vi "DSF.Engine.Runtime.Plugin.Get ID.vi"(8 "error in (no error)":errorcluster, 11 "Plugin in":refnum<class "DSF.Engine.Runtime.Plugin.lvclass">) -> (0 "error out":errorcluster, 2 "id":i32, 3 "Plugin out":refnum<class "DSF.Engine.Runtime.Plugin.lvclass">)   [LabVIEW 2016, in "DSF.Engine.lvlib" / "DSF.Engine.Runtime.Plugin.lvclass"]
uses:
  DSF.Engine.Runtime.Plugin.lvclass
  DSF.Engine.Runtime.Plugin.lvclass/DSF.Engine.Runtime.Plugin.ctl
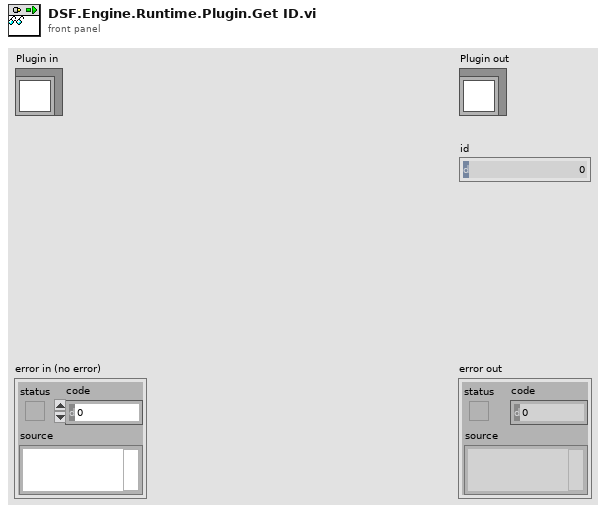
[diagram p1: front panel]
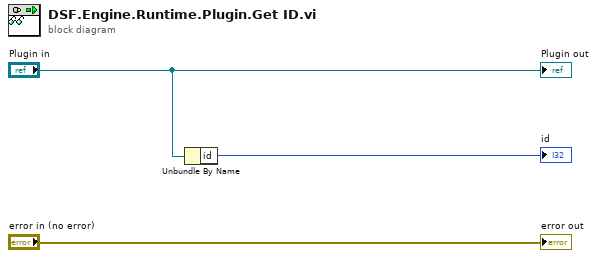
[diagram p0: block diagram]
diagram:
  n1 = Unbundle By Name("Plugin in") -> ("id"=→"id":i32)
  "error out" <- "error in (no error)"
  "Plugin out" <- "Plugin in"
